vi "_editDialog.vi"(0 "reference":refnum<class "InitialStateNode.lvclass">, 1 "insidePackageNode":bool, 5 "error in (no error)":errorcluster) -> (14 "reference out":refnum<class "InitialStateNode.lvclass">, 15 "changeConnection":T1, 16 "cancel":bool, 19 "error out":errorcluster)   [LabVIEW 2014, in "InitialStateNode.lvclass"]
doc: "Edit Dialog"
uses:
  <resource>/Framework/Providers/Open_GDS/UML/InitialStateNode_class/InitialStateNode.lvclass
  <resource>/Framework/Providers/Open_GDS/UML/AbstractNode_class/private/NodeConnectionStatsType.ctl
  <resource>/Framework/Providers/Open_GDS/UML/ContextHelp/ContextHelp_HelpTexts.ctl
  <resource>/Framework/Providers/Open_GDS/UML/MultiLineString_class/MultiLineString.lvclass
  <resource>/Framework/Providers/Open_GDS/UML/AbstractNode_class/AbstractNode.lvclass
panel:
  in  "OK Button":bool
  in  "Cancel Button":bool
  in  "Help":bool
  in  "connection":bool caption="Connect to System"
  in  "Initial text":string
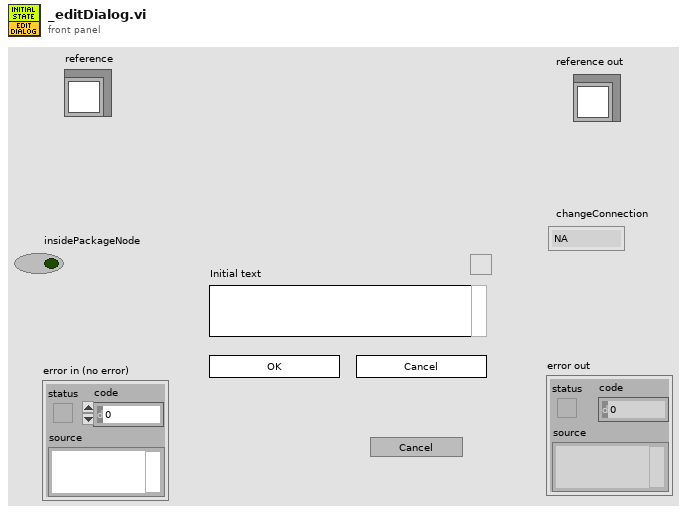
[diagram p1: front panel]
types:
  T1 = typedef "AbstractNode.lvclass/NodeConnectionStatsType.ctl" = enum16{"NA", "Connect", "DisConnect"}
  T2 = typedef "ContextHelp_HelpTexts.ctl" = enum16{"None(Hide)", "Default", "Help", "Welcome", "GettingStarted", "ClassDiagram_Help", "SequenceDiagram_Help", "UseCaseDiagram_Help", "BSelect", "BClass", "BInterface", "BPackage", "BNote", "BDependency", "BInheritance", "BInterfaceImplementation", "BAssociation", "BAggregation", "BCompAggregation", "BNoteConnector", "BObject", "BActionBar", "BCall", "BSystem", "BActor", "BUseCase", "BGeneralization", "BIncludes", "BExtends", "BUseCaseDiagramAssociation", "ClassRelationshipEdge editDialog_Bent Style", "ClassRelationshipEdge editDialog_RelationType", "ClassRelationshipEdge editDialog_Reverse association", "ClassRelationshipEdge editDialog_Start label", "ClassRelationshipEdge editDialog_Middle label", "ClassRelationshipEdge editDialog_End label", "UMLEditor reversedEngineering_Pathes", "ReversedEngineering StateReverseDialog_Help", "ReversedEngineering StateQueuedSettings_Help", "UMLEditor reversedEngineering_AddTopVIs", "UMLEditor reversedEngineering_AddClasses", "UMLEditor reversedEngineering_AddDirs", "UMLEditor reversedEngineering_Recursively", "UMLEditor reversedEngineering_Remove", "UMLEditor reversedEngineering_ClearList", "UMLEditor reversedEngineering_HideSubAss", "UMLEditor reversedEngineering_CreateTypes", "UMLEditor reversedEngineering_OnlyInheritance", "UMLEditor reversedEngineering_CreateApplication", "UMLEditor reversedEngineering_OK", "UMLEditor reversedEngineering_Cancel", "UMLEditor reversedEngineering_Help", "UMLEditor createWizardScriptFile_ScriptfilePath", "UMLEditor createWizardScriptFile_ClassPath", "UMLEditor createWizardScriptFile_Use", "UMLEditor createWizardScriptFile_PrivateDirName", "UMLEditor createWizardScriptFile_DirAppend", "UMLEditor createWizardScriptFile_Separator Character", "UMLEditor createWizardScriptFile_OK", "UMLEditor createWizardScriptFile_Cancel", "UMLEditor createWizardScriptFile_Help", "ClassNode editDialog_Class Name", "InterfaceNode editDialog_Class Name", "ClassNode editDialog_Attribute", "ClassNode editDialog_Methods", "InterfaceNode editDialog_Methods", "ClassNode editDialog_connection", "InterfaceNode editDialog_connection", "ClassNode editDialog_StereoType", "ClassNode editDialog_ShowAttrib", "ClassNode editDialog_ShowMethods", "ClassNode editDialog_ClassPath", "ClassNode editDialog_AddAttribute", "ClassNode editDialog_AddMethod", "InterfaceNode editDialog_AddMethod", "ClassNode AttributeGuide_AttributeName", "ClassNode AttributeGuide_Array?", "ClassNode AttributeGuide_Data Type", "ClassNode AttributeGuide_RefName", "ClassNode AttributeGuide_Preview", "ClassNode AttributeGuide_OK", "ClassNode AttributeGuide_Cancel", "ClassNode MethodGuide_Visibility", "ClassNode MethodGuide_Method Name", "ClassNode MethodGuide_Preview", "ClassNode MethodGuide_OK", "ClassNode MethodGuide_Cancel", "CallNode EditCallProperties_AllButtons", "ObjectNode EditObjectlProperties_AllButtons", "ActorNode EditActorProperties_AllButtons", "UseCaseRelationshipNode EditUseCaselProperties_AllButtons", "UseCaseNode EditUseCaselProperties_AllButtons", "SystemNode EditSystemProperties_AllButtons", "ReversedEngineering UpdateAttributes_AllButtons", "StateNode editDialog_AllButtons", "StateTransition editDialog_AllButtons", "ArrangeNodes Main_Picture", "ArrangeNodes Main_Zoom", "ArrangeNodes Main_Auto Zoom", "ArrangeNodes Main_shorten", "ArrangeNodes Main_Min Length", "ArrangeNodes Main_Max Length", "ArrangeNodes Main_increase", "ArrangeNodes Main_decrease", "ArrangeNodes Main_Shake", "ArrangeNodes Main", "BState", "BInitialState", "BFinalState", "BStateTransition", "StateDiagram_Help", "StateDiagram_PropertiesAllButtons", "ReversedEngineering StateReverseDialog_ClearStates", "ReversedEngineering StateReverseDialog_UseQueuedStateMachines", "ReversedEngineering StateReverseDialog_QueuedSettings", "ReversedEngineering StateReverseDialog_SearchForVIs", "ReversedEngineering StateReverseDialog_SearchCriteria", "OptionsDialog_ClassBasePath", "OptionsDialog_VIPath", "OptionsDialog_ApplicationPath", "OptionsDialog_WizDir", "OptionsDialog_IniFilePath", "OptionsDialog_DefineColors", "OptionsDialog_Help", "OptionsDialog_CreateTypes", "ClassRelationshipEdge editDialog_SplitWire"}
  T3 = typedef "InitialStateNode.lvclass/ObjectAttributes.ctl" = cluster{"Base class":T4, "name":refnum<class "MultiLineString.lvclass">, "DEFAULT_WIDTH":i32, "DEFAULT_HEIGHT":i32}
  T4 = typedef "RectangularNode.lvclass/ObjectAttributes.ctl" = cluster{"Base class":T5, "bounds":T6}
  T5 = typedef "AbstractNode.lvclass/ObjectAttributes.ctl" = cluster{"parent":refnum<class "AbstractNode.lvclass">, "children":refnum<class "AbstractNode.lvclass">[], "Hidden":bool}
  T6 = typedef "Rectangle Rectangle2D.ctl" = cluster{"x":dbl, "y":dbl, "width":dbl, "height":dbl}
  T7 = typedef "ContextHelp_ShowType.ctl" = cluster{"Header":string, "Picture":picture, "Text":string}
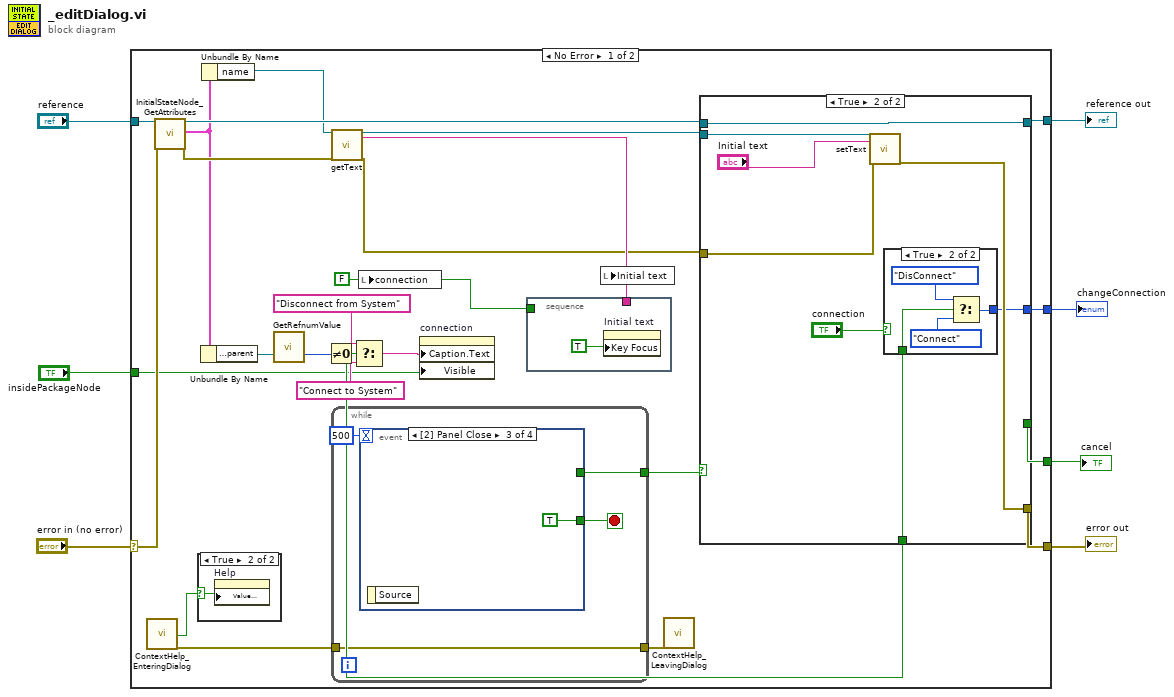
[diagram p0: block diagram]
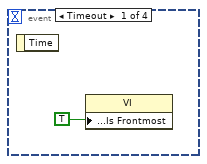
[diagram p3: hidden frame]
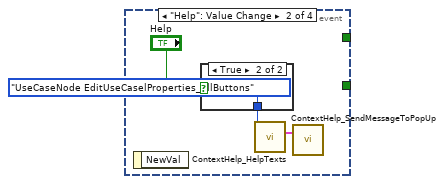
[diagram p4: hidden frame]
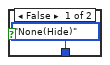
[diagram p5: hidden frame]
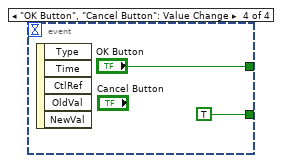
[diagram p6: hidden frame]
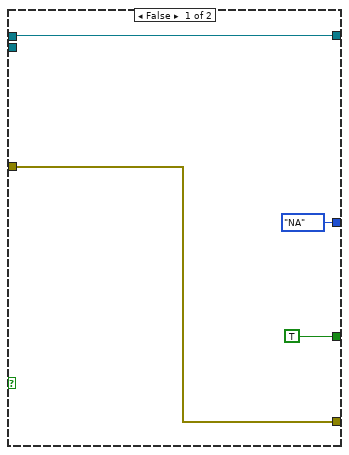
[diagram p7: hidden frame]
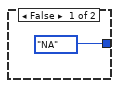
[diagram p8: hidden frame]
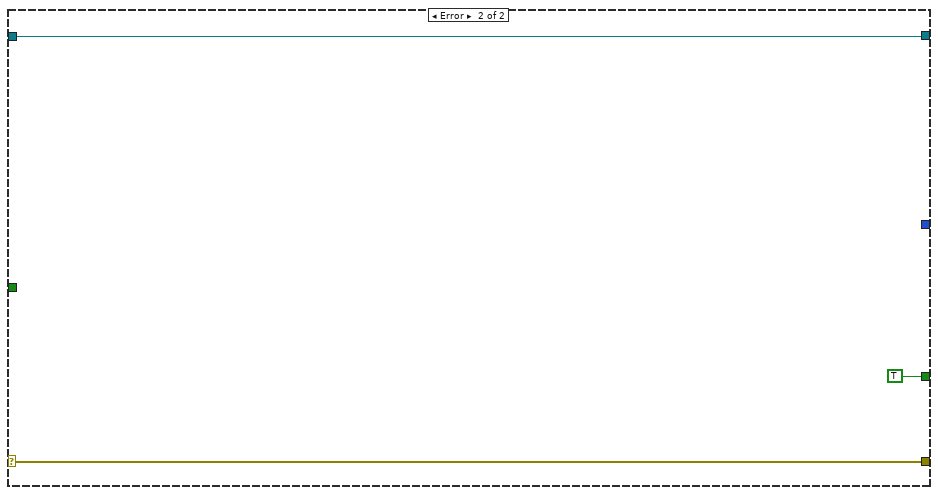
[diagram p9: hidden frame]
diagram:
  n1 = case shown="No Error" "error in (no error)" {
    selector: "error in (no error)" -> [w28 w66]
    tunnel: "reference" -> [w29 w67]
    tunnel: [w32 w66] -> w5
    tunnel: [w31 w67] -> w4
    tunnel: [w23 _] -> w3
    tunnel: "insidePackageNode" -> [w17 _]
    tunnel: [w15 TRUE ("Key Focus")] -> w1
    frame No Error {
      w16 = FALSE ("connection")
      n2 = call <resource>:"ContextHelp_EnteringDialog.vi"() -> ("HelpStatus"=w10:bool, "error out"=w12:errorcluster)  [unwired: 3 in, 15 out]
      n3 = call <resource>:"InitialStateNode_GetAttributes.vi"("reference in"=w29, "error in (no error)"=w28) -> ("reference out"=w30:refnum<class "InitialStateNode.lvclass">, "Attributes"=w18:T3, "error out"=w27:errorcluster)  [unwired: 15 out]
      n4 = case shown="True" w10 {
        selector: w10 -> [_ w33]
        frame False {
        }
        frame True {
          n5 = property on="Help" class="Bool (strict)"("Value (Signaling)"=w33) -> ()  [unwired: 2 in, 2 out]
        }
      }
      n6 = Unbundle By Name(w18) -> ("Base class.Base class.parent"=w9:refnum<class "AbstractNode.lvclass">)
      n7 = Unbundle By Name(w18) -> ("name"=w24:refnum<class "MultiLineString.lvclass">)
      n8 = call <resource>:"GetRefnumValue.vi"("reference"=w9) -> ("RefNum"=w8:i32)  [unwired: 17 in, 1 out]
      n9 = Not Equal To 0?(x=w8) -> (x != 0?=w22:bool)
      n10 = call-dynamic "getText.vi"("reference"=w24, "error in (no error)"=w27) -> ("reference out"=w26:refnum<class "MultiLineString.lvclass">, "text"=w25:string, "error out"=w14:errorcluster)  [unwired: 15 in]
      n11 = while {
        tunnel: [w37] -> w11
        tunnel: [w35] -> w13
        tunnel: w12 -> [w35]
        stop <- w36 stop-if-true
        n12 = event shown="[2] Panel Close" {
          selector: _ -> [_ _ _ _]
          dyn-events: _ -> [_ _ _ _]
          timeout: 500 -> [_ _ _ _]
          tunnel: [_ _ _ "OK Button"] -> w37
          tunnel: [_ _ TRUE TRUE] -> w36
          event Timeout {
            n13 = event-data() -> ()  [unwired: 2 out]
            n14 = property class="VI"("Front Panel Window:Is Frontmost"=TRUE) -> ()  [unwired: 2 in, 2 out]
          }
          event "Help": Value Change {
            n15 = event-data() -> ()  [unwired: 2 out]
            n16 = case shown="True" "Help" {
              tunnel: [ContextHelp_HelpTexts."None(Hide)" ("HelpText") ContextHelp_HelpTexts."UseCaseNode EditUseCaselProperties_AllButtons" ("HelpText")] -> w40
              frame False {
              }
              frame True {
              }
            }
            n17 = call <resource>:"ContextHelp_HelpTexts.vi"("HelpText (enum or string)"=w40) -> ("HelpOut"=w41:T7)  [unwired: 18 out]
            n18 = call <resource>:"ContextHelp_SendMessageToPopUp.vi"("PopUpMessage"=w41) -> ()  [unwired: 2 in, 17 out]
          }
          event Panel Close {
            n19 = event-data() -> ()  [unwired: 2 out]
          }
          event "OK Button", "Cancel Button": Value Change {
            n20 = event-data() -> ()  [unwired: 6 out]
          }
        }
      }
      n21 = Select(t="Disconnect from System", s=w22, f="Connect to System") -> (s? t:f=w21:string)
      n22 = local write "connection"(w16) -> ()
      n23 = property on="connection" class="Bool (strict)"("Caption.Text"=w21, "Visible"=w17) -> ()  [unwired: 2 in, 2 out]
      n24 = stacked-sequence {
        tunnel: w25 -> [_]
        tunnel: w16 -> [_]
        frame #0 {
          n25 = property on="Initial text" class="Str"("Key Focus"=TRUE) -> ()  [unwired: 2 in, 2 out]
        }
      }
      n26 = local write "Initial text"(w25) -> ()
      n27 = call <resource>:"ContextHelp_LeavingDialog.vi"("error in (no error)"=w13) -> ()  [unwired: 2 in, 17 out]
      n28 = case shown="True" w11 {
        tunnel: [w49 w55] -> w32
        tunnel: [w50 w56] -> w31
        tunnel: w30 -> [w50 w56]
        tunnel: w26 -> [_ w58]
        tunnel: w14 -> [w49 w51]
        tunnel: [enum16{"NA", "Connect", "DisConnect"}."NA" ("changeConnection") w53] -> w23
        tunnel: w22 -> [_ w52]
        tunnel: [TRUE ("Key Focus") _] -> w15
        frame False {
        }
        frame True {
          n29 = call-dynamic "setText.vi"("reference"=w58, "text"="Initial text", "error in (no error)"=w51) -> ("error out"=w55:errorcluster)  [unwired: 15 in, 1 out]
          n30 = case shown="True" "connection" {
            tunnel: [enum16{"NA", "Connect", "DisConnect"}."NA" ("changeConnection") w62] -> w53
            tunnel: w52 -> [_ w63]
            frame False {
            }
            frame True {
              n31 = Select(t=enum16{"NA", "Connect", "DisConnect"}."DisConnect" ("changeConnection"), s=w63, f=enum16{"NA", "Connect", "DisConnect"}."Connect" ("changeConnection")) -> (s? t:f=w62:enum16{"NA", "Connect", "DisConnect"})
            }
          }
        }
      }
    }
    frame Error {
    }
  }
  "reference out" <- w4
  "error out" <- w5
  "changeConnection" <- w3
  "cancel" <- w1
